vi "Close XML.vi"(8 "error in (no error)":errorcluster, 11 "DOM document in":refnum<k20>) -> (0 "error out":errorcluster)   [LabVIEW 2016, in "SLL File IO.lvlib"]
doc: "Closes the XML reference."
uses:
  SLL File IO.lvlib
  <vilib>/xml/Close Reference(Node).vi
  <vilib>/xml/NI_XML.lvlib
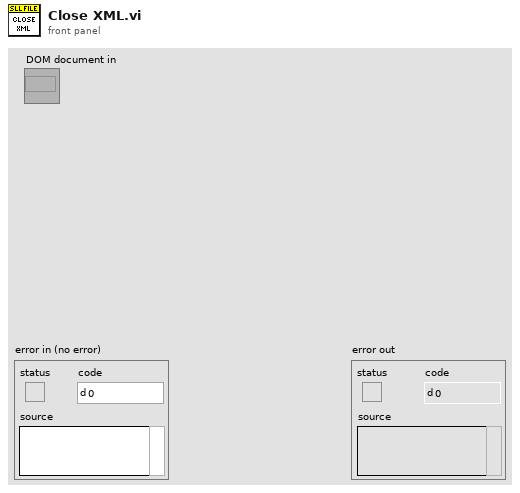
[diagram p1: front panel]
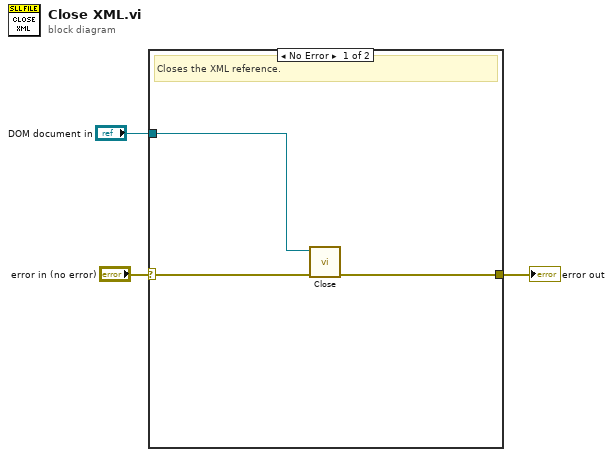
[diagram p0: block diagram]
diagram:
  n1 = case shown="No Error" "error in (no error)" {
    selector: "error in (no error)" -> [w6 w7]
    tunnel: [w5 w7] -> w2
    tunnel: "DOM document in" -> [w4 _]
    frame No Error {
      # "Closes the XML reference."
      n2 = call-poly <vilib>:"Close.vi"("error in (no error)"=w6, "node"=w4) -> ("error out"=w5:errorcluster)  [unwired: 7 in]
    }
    frame Error {
    }
  }
  "error out" <- w2
